vi "Subspaces Angle (2D).vi"(10 "B":T1, 11 "A":T1) -> (0 "error":i32, 3 "angle":dbl)   [LabVIEW 2017, in "NI_AAL_LinAlg.lvlib"]
doc: "Computes the angle between column spaces of two matrices."
uses:
  <vilib>/Analysis/NI_AAL_LinAlg.lvlib
  <vilib>/Analysis/Matrix/Datatypes/RealMatrix.ctl
  <vilib>/Analysis/7linalg.llb/SVD Option.ctl
  <vilib>/Analysis/baseanly.llb/Real A x B.vi
  <vilib>/Analysis/_algsub.llb/Real Matrix Norm.vi
  <vilib>/Analysis/7linalg.llb/Real SVD Decomposition.vi
  <vilib>/Analysis/Matrix/Numeric/Subtract/Subtract - RM,RM.vi
  <vilib>/Analysis/NI_AALBase.lvlib
  <vilib>/Analysis/NI_AALPro.lvlib
  <vilib>/Analysis/Matrix/NI_Matrix.lvlib
panel:
  # "Angle Between Subspaces (2D)"
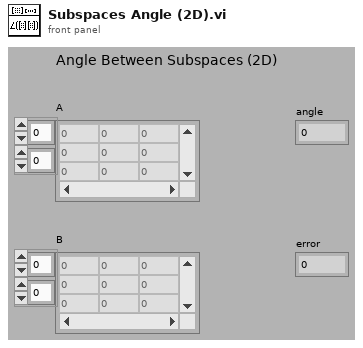
[diagram p1: front panel]
types:
  T1 = typedef "NI_Matrix.lvlib/RealMatrix.ctl" = dbl[][]
  T2 = typedef "NI_AALPro.lvlib/SVD Option.ctl" = u16
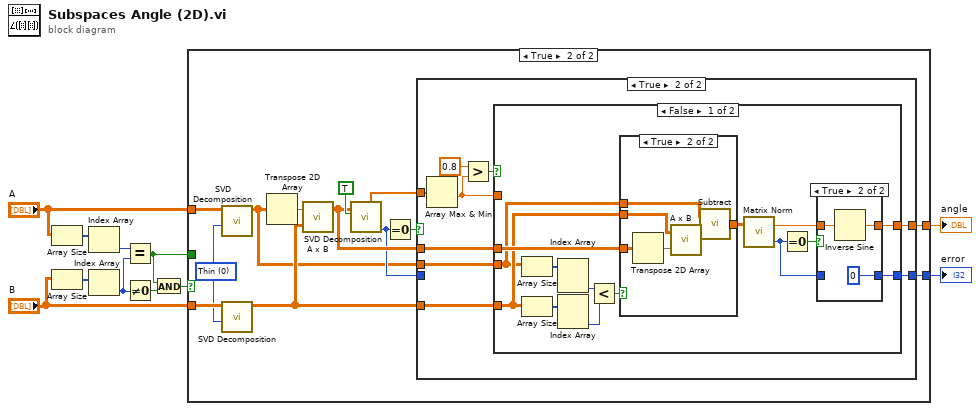
[diagram p0: block diagram]
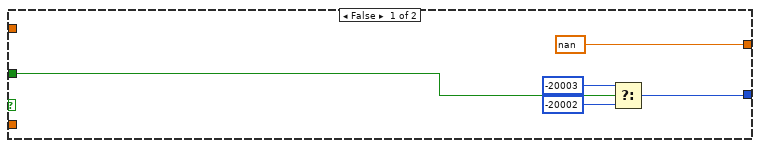
[diagram p2: hidden frame]
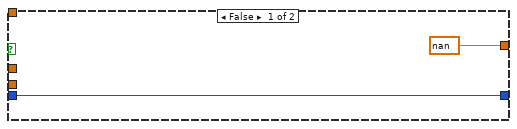
[diagram p3: hidden frame]
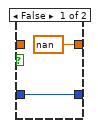
[diagram p4: hidden frame]
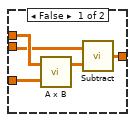
[diagram p5: hidden frame]
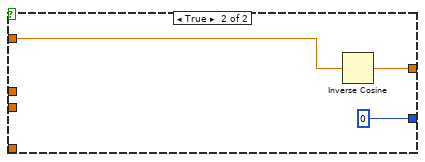
[diagram p6: hidden frame]
diagram:
  n1 = Array Size(array="A") -> (size(s)=w11:i32[])
  n2 = Array Size(array="B") -> (size(s)=w10:i32[])
  n3 = Index Array(array=w11) -> (element=w9:i32)  [unwired: 1 in]
  n4 = Index Array(array=w10) -> (element=w4:i32)  [unwired: 1 in]
  n5 = Equal?(x=w9, y=w4) -> (x = y?=w1:bool)
  n6 = Not Equal To 0?(x=w4) -> (x != 0?=w3:bool)
  n7 = And(x=w1, y=w3) -> (x .and. y?=w2:bool)
  n8 = case shown="True" w2 {
    tunnel: "A" -> [_ w29]
    tunnel: "B" -> [_ w28]
    tunnel: [nan w25] -> w8
    tunnel: [w13 w21] -> w7
    tunnel: w1 -> [w15 _]
    frame False {
      n9 = Select(t=-20003, s=w15, f=-20002) -> (s? t:f=w13:i32)
    }
    frame True {
      w17 = T2 0 items=["Thin", "Full"] ("SVD option")
      n10 = call-poly <vilib>:"SVD Decomposition.vi"("SVD option"=w17, "A"=w29) -> ("Matrix U"=w19:T1)  [unwired: 1 in, 8 out]
      n11 = call-poly <vilib>:"SVD Decomposition.vi"("SVD option"=w17, "A"=w28) -> ("Matrix U"=w23:T1)  [unwired: 1 in, 8 out]
      n12 = Transpose 2D Array(2D array=w19) -> (transposed array=w18:T1)
      n13 = call-poly <vilib>:"A x B.vi"("B"=w23, "A"=w18) -> ("A x B"=w24:T1)  [unwired: 1 out]
      n14 = call-poly <vilib>:"SVD Decomposition.vi"("singular values only?"=TRUE, "A"=w24) -> ("error"=w20:i32, "Vector S"=w26:dbl[])  [unwired: 1 in, 7 out]
      n15 = Equal To 0?(x=w20) -> (x = 0?=w22:bool)
      n16 = case shown="True" w22 {
        tunnel: w26 -> [_ w40]
        tunnel: [nan w37] -> w25
        tunnel: w19 -> [_ w36]
        tunnel: w24 -> [_ w35]
        tunnel: w23 -> [_ w34]
        tunnel: [w31 w33] -> w21
        tunnel: w20 -> [w31 _]
        frame False {
        }
        frame True {
          n17 = Array Max & Min(array=w40) -> (min value=w38:dbl)  [unwired: 3 out]
          n18 = Greater?(x=0.8 ("threshold"), y=w38) -> (0:w39:bool)
          n19 = case shown="False" w39 {
            tunnel: [w51 w72] -> w37
            tunnel: w38 -> [_ w71]
            tunnel: w36 -> [w41 _]
            tunnel: w34 -> [w42 _]
            tunnel: w35 -> [w48 _]
            tunnel: [w46 0 ("error")] -> w33
            frame False {
              n20 = Array Size(array=w41) -> (size(s)=w49:i32[])
              n21 = Array Size(array=w42) -> (size(s)=w50:i32[])
              n22 = Index Array(array=w49) -> (element #2=w44:i32)  [unwired: 2 in, 1 out]
              n23 = Index Array(array=w50) -> (element #2=w43:i32)  [unwired: 2 in, 1 out]
              n24 = Less?(x=w44, y=w43) -> (x < y?=w54:bool)
              n25 = case shown="True" w54 {
                tunnel: w42 -> [w61 w68]
                tunnel: [w64 w70] -> w53
                tunnel: w48 -> [w62 w67]
                tunnel: w41 -> [w63 w69]
                frame False {
                  n26 = call-poly <vilib>:"A x B.vi"("B"=w62, "A"=w63) -> ("A x B"=w60:T1)  [unwired: 1 out]
                  n27 = call-poly <vilib>:"Subtract.vi"("Real Matrix B"=w60, "Real Matrix A"=w61) -> ("A - B"=w64:T1)
                }
                frame True {
                  n28 = Transpose 2D Array(2D array=w67) -> (transposed array=w66:T1)
                  n29 = call-poly <vilib>:"A x B.vi"("B"=w66, "A"=w68) -> ("A x B"=w65:T1)  [unwired: 1 out]
                  n30 = call-poly <vilib>:"Subtract.vi"("Real Matrix B"=w65, "Real Matrix A"=w69) -> ("A - B"=w70:T1)
                }
              }
              n31 = call-poly <vilib>:"Matrix Norm.vi"("Input Matrix"=w53) -> ("error"=w45:i32, "norm"=w52:dbl)  [unwired: 1 in]
              n32 = Equal To 0?(x=w45) -> (x = 0?=w47:bool)
              n33 = case shown="True" w47 {
                tunnel: w52 -> [_ w58]
                tunnel: [nan w57] -> w51
                tunnel: [w56 0 ("error")] -> w46
                tunnel: w45 -> [w56 _]
                frame False {
                }
                frame True {
                  n34 = Inverse Sine(1:w58) -> (0:w57:dbl)
                }
              }
            }
            frame True {
              n35 = Inverse Cosine(1:w71) -> (0:w72:dbl)
            }
          }
        }
      }
    }
  }
  "angle" <- w8
  "error" <- w7
